vi "Polling Wait.vi"(8 "error in (no error)":errorcluster, 11 "seconds to wait":dbl format="%#_6p") -> (0 "error out":errorcluster)   [LabVIEW 2022 SP3]
uses:
  RT Sub VI's/RT Global.vi
  kernel32.dll
panel:
  out "done":bool
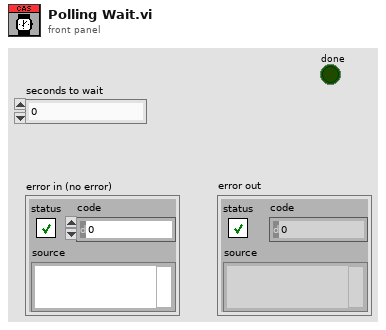
[diagram p1: front panel]
types:
  T1 = cluster{"time_t seconds":i64, "int nanoseconds":i32}
  T2 = cluster{"time_t seconds":i32, "int nanoseconds":i32}
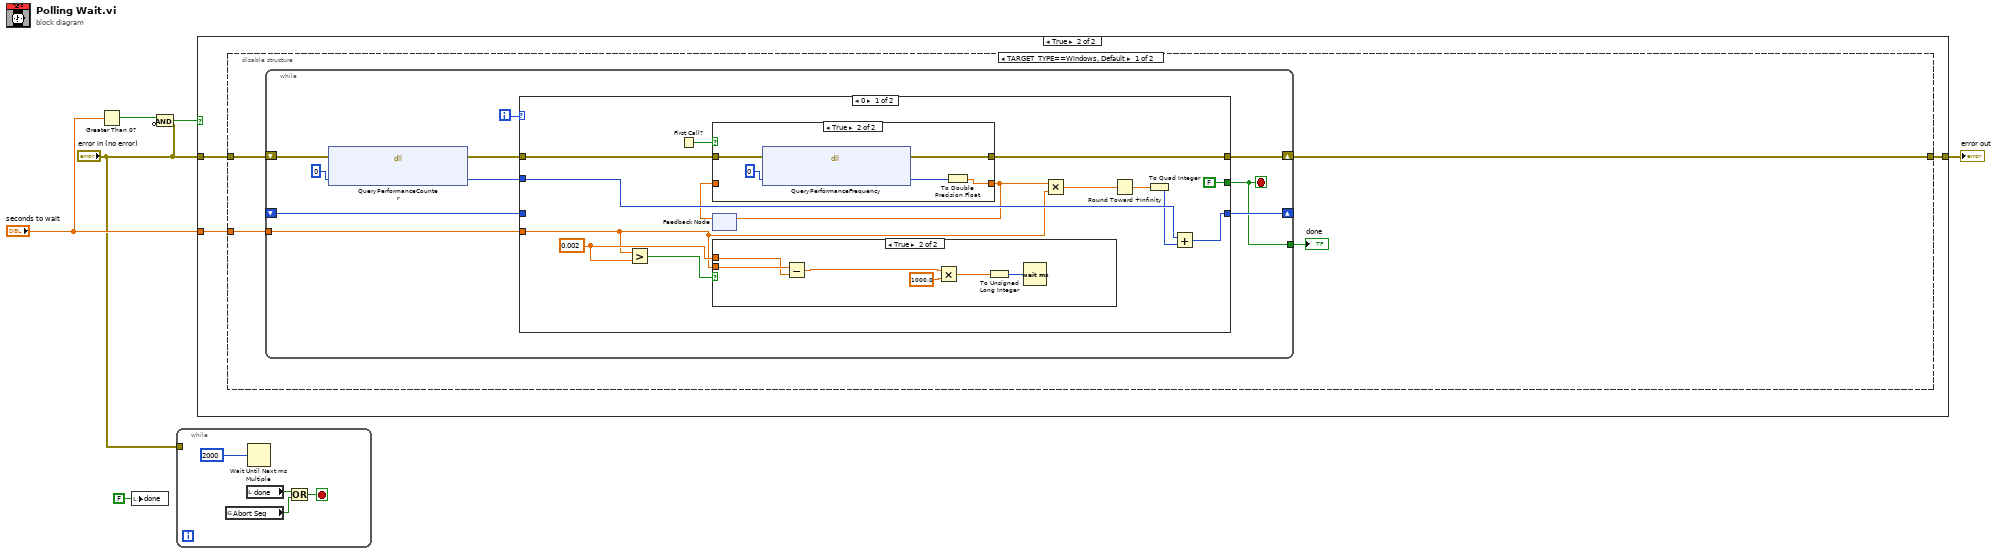
[diagram p0: block diagram]
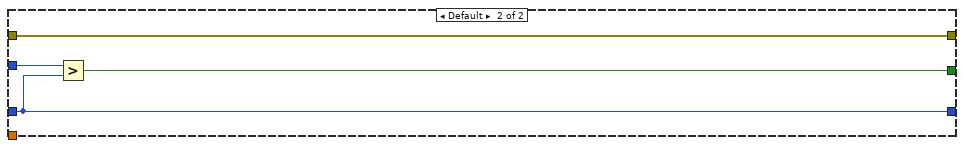
[diagram p5: hidden frame]
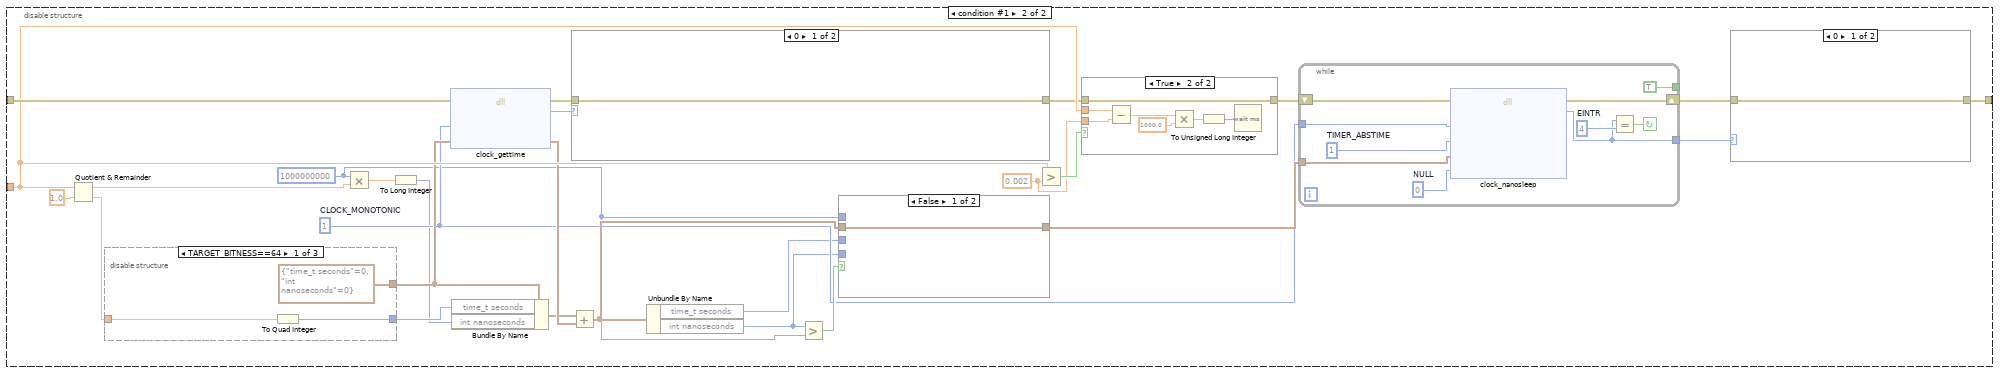
[diagram p6: hidden frame]
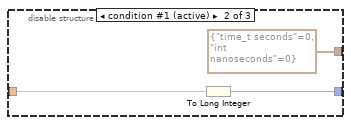
[diagram p7: hidden frame]
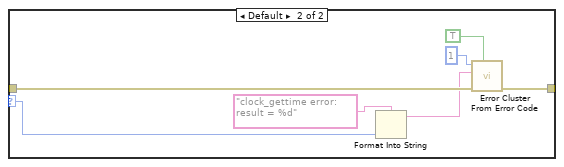
[diagram p10: hidden frame]
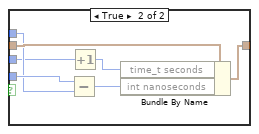
[diagram p11: hidden frame]
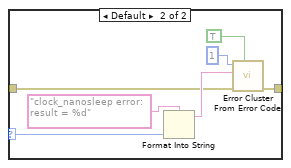
[diagram p12: hidden frame]
diagram:
  n1 = Greater Than 0?(x="seconds to wait") -> (x > 0?=w4:bool)
  n2 = local write "done"(FALSE ("done")) -> ()
  n3 = Compound Arithmetic op=AND(w4, invert "error in (no error)") -> (w3:bool)
  n4 = while {
    tunnel: "error in (no error)" -> [_]
    stop <- w8 stop-if-true
    n5 = global read "RT Global.vi" "Abort Seq"() -> (w9:bool)
    n6 = local read "done"() -> (w7:bool)
    n7 = Wait Until Next ms Multiple(millisecond multiple=u32 2000) -> ()  [unwired: 1 out]
    n8 = Or(x=w7, y=w9) -> (x .or. y?=w8:bool)
  }
  n9 = case shown="True" w3 {
    tunnel: "seconds to wait" -> [_ w14]
    tunnel: [w11 w12] -> w6
    tunnel: "error in (no error)" -> [w11 w13]
    frame False {
    }
    frame True {
      n10 = disable-structure shown="TARGET_TYPE==Windows, Default" {
        disable-tunnel: w14 -> [w18 w82]
        disable-tunnel: w13 -> [w17 w86]
        disable-tunnel: [w16 w84] -> w12
        frame condition #0 (active) {
          n11 = while {
            shift-right: [w27] -> _
            shift-left: _ -> [w28]
            tunnel: w18 -> [w25]
            shift-right: [w21] -> w16
            shift-left: w17 -> [w23]
            tunnel: [w19] -> w15
            i -> [w26]
            stop <- w19 stop-if-true
            n12 = dll-call lib="kernel32.dll" fn="QueryPerformanceCounter"(error in=w23, "lpPerformanceCount"=i64 0) -> (error out=w22:errorcluster, "lpPerformanceCount"=w24:i64)  [unwired: 3 in, 1 out]
            n13 = case shown="0" w26 {
              tunnel: w28 -> [_ w58]
              tunnel: [w42 w58] -> w27
              tunnel: [FALSE w59] -> w19
              tunnel: w25 -> [w34 _]
              tunnel: w24 -> [w38 w57]
              tunnel: w22 -> [w30 w56]
              tunnel: [w29 w56] -> w21
              frame 0 {
                w39 = 0.002 ("y")
                n14 = Greater?(x=w34, y=w39) -> (0:w40:bool)
                n15 = First Call?() -> (First Call?: T/F=w33:bool)
                n16 = feedback #1() -> (w31:dbl)  [unwired: 1 in]
                n17 = case shown="True" w33 {
                  tunnel: w31 -> [w44 _]
                  tunnel: [w44 w49] -> w32
                  tunnel: w30 -> [w43 w48]
                  tunnel: [w43 w47] -> w29
                  frame False {
                  }
                  frame True {
                    n18 = dll-call lib="kernel32.dll" fn="QueryPerformanceFrequency"(error in=w48, "lpFrequency"=i64 0) -> (error out=w47:errorcluster, "lpFrequency"=w46:i64)  [unwired: 3 in, 1 out]
                    n19 = To Double Precision Float(number=w46) -> (double precision float=w49:dbl)
                  }
                }
                n20 = feedback-in #1(w32) -> ()
                n21 = case shown="True" w40 {
                  tunnel: w34 -> [_ w51]
                  tunnel: w39 -> [_ w50]
                  frame False {
                  }
                  frame True {
                    n22 = Subtract(x=w51, y=w50) -> (x-y=w55:dbl)
                    n23 = Multiply(x=w55, y=1000.0) -> (x*y=w52:dbl)
                    n24 = To Unsigned Long Integer(number=w52) -> (unsigned 32bit integer=w53:u32)
                    n25 = Wait (ms)(milliseconds to wait=w53) -> ()  [unwired: 1 out]
                  }
                }
                n26 = Multiply(x=w32, y=w34) -> (x*y=w37:dbl)
                n27 = Round Toward +Infinity(x=w37) -> (ceil(x): smallest int >= x=w36:dbl)
                n28 = To Quad Integer(1:w36) -> (0:w35:i64)
                n29 = Add(x=w38, y=w35) -> (x+y=w42:i64)
              }
              frame Default {
                n30 = Greater?(x=w57, y=w58) -> (0:w59:bool)
              }
            }
          }
          "done" <- w15
        }
        frame condition #1 {
          w64 = 0.002 ("y")
          w71 = 1  # CLOCK_MONOTONIC
          w69 = 1000000000 ("x")
          n31 = Quotient & Remainder(x=w82, y=1.0) -> (x-y*floor(x/y)=w61:dbl, floor(x/y)=w80:dbl)
          n32 = disable-structure shown="TARGET_BITNESS==64" {
            disable-tunnel: w80 -> [w89 w92 _]
            disable-tunnel: [T1 {"time_t seconds"=0, "int nanoseconds"=0} ("timespec type") T2 {"time_t seconds"=0, "int nanoseconds"=0} ("timespec type") _] -> w79
            disable-tunnel: [w87 w90 _] -> w73
            frame condition #0 {
              n33 = To Quad Integer(1:w89) -> (0:w87:i64)
            }
            frame condition #1 (active) {
              n34 = To Long Integer(number=w92) -> (32bit integer=w90:i32)
            }
            frame condition #2 {
              # "Break if we're not\n32 or 64 bits."
            }
          }
          n35 = Multiply(x=w69, y=w61) -> (x*y=w72:dbl)
          n36 = To Long Integer(number=w72) -> (32bit integer=w60:i32)
          n37 = dll-call lib="LabVIEW" fn="clock_gettime"(error in=w86, "clock_id"=w71, "timespecPtr_time"=w79) -> (error out=w67:errorcluster, "result"=w66:i32, "timespecPtr_time"=w78:T2)  [unwired: 3 in, 1 out]
          n38 = Bundle By Name(cluster=w79, "time_t seconds"=w73, "int nanoseconds"=w60) -> (w76:T2)
          n39 = Add(x=w76, y=w78) -> (x+y=w75:T2)
          n40 = case shown="0" w66 {
            selector: w66 -> [_ w103]
            tunnel: w67 -> [w101 w105]
            tunnel: [w101 w108] -> w63
            frame 0 {
            }
            frame Default {
              n41 = Format Into String(format string="clock_gettime error: result = %d", w103) -> (resulting string=w104:string)  [unwired: 2 in, 1 out]
              n42 = call <vilib>:"Error Cluster From Error Code.vi"("show call chain? (False)"=TRUE, "error in (no error)"=w105, "error message (\"\")"=w104, "error code (0)"=1) -> ("error out"=w108:errorcluster)  [unwired: 5 in]
            }
          }
          n43 = Unbundle By Name(w75) -> ("time_t seconds"=w68:i32, "int nanoseconds"=w70:i32)
          n44 = Greater?(x=w70, y=w69) -> (0:w77:bool)
          n45 = case shown="False" w77 {
            tunnel: [w119 w126] -> w74
            tunnel: w75 -> [w119 w125]
            tunnel: w70 -> [_ w124]
            tunnel: w69 -> [_ w123]
            tunnel: w68 -> [_ w122]
            frame False {
            }
            frame True {
              n46 = Subtract(x=w124, y=w123) -> (x-y=w120:i32)
              n47 = Increment(x=w122) -> (x+1=w121:i32)
              n48 = Bundle By Name(cluster=w125, "time_t seconds"=w121, "int nanoseconds"=w120) -> (w126:T2)
            }
          }
          n49 = Greater?(x=w82, y=w64) -> (0:w65:bool)
          n50 = case shown="True" w65 {
            tunnel: w82 -> [_ w96]
            tunnel: w64 -> [_ w95]
            tunnel: w63 -> [w93 w94]
            tunnel: [w93 w94] -> w62
            frame False {
            }
            frame True {
              n51 = Subtract(x=w96, y=w95) -> (x-y=w100:dbl)
              n52 = Multiply(x=w100, y=1000.0) -> (x*y=w97:dbl)
              n53 = To Unsigned Long Integer(number=w97) -> (unsigned 32bit integer=w98:u32)
              n54 = Wait (ms)(milliseconds to wait=w98) -> ()  [unwired: 1 out]
            }
          }
          n55 = while {
            tunnel: w74 -> [w116]
            shift-right: [w118] -> w85
            shift-left: w62 -> [w117]
            tunnel: w71 -> [w111]
            tunnel: [w110] -> w83
            tunnel: [TRUE] -> _
            stop <- w114 continue-if-true
            w112 = u64 0  # NULL
            w113 = 1  # TIMER_ABSTIME
            w115 = 4  # EINTR
            n56 = dll-call lib="LabVIEW" fn="clock_nanosleep"(error in=w117, "clock_id"=w111, "flags"=w113, "timespecPtr_request"=w116, "timespecPtr_remainder"=w112) -> (error out=w118:errorcluster, "result"=w110:i32)  [unwired: 6 in, 1 out]
            n57 = Equal?(x=w110, y=w115) -> (x = y?=w114:bool)
          }
          n58 = case shown="0" w83 {
            selector: w83 -> [_ w128]
            tunnel: w85 -> [w127 w130]
            tunnel: [w127 w129] -> w84
            frame 0 {
            }
            frame Default {
              n59 = Format Into String(format string="clock_nanosleep error: result = %d", w128) -> (resulting string=w132:string)  [unwired: 2 in, 1 out]
              n60 = call <vilib>:"Error Cluster From Error Code.vi"("show call chain? (False)"=TRUE, "error in (no error)"=w130, "error message (\"\")"=w132, "error code (0)"=1) -> ("error out"=w129:errorcluster)  [unwired: 5 in]
            }
          }
        }
      }
    }
  }
  "error out" <- w6
